vi "Request API.vi"(8 "error in (no error)":errorcluster, 10 "Promise":refnum<class "Promise.lvclass">, 11 "API Provider in":refnum<class "API Provider.lvclass">) -> (0 "error out":errorcluster, 3 "API Provider out":refnum<class "API Provider.lvclass">)   [LabVIEW 2020, in "Volatus.lvlib" / "API Provider.lvclass"]
uses:
  API Provider.lvclass
  lv-promises/Promises/Promise/Promise.lvclass
  ApiValue/ApiValue.lvclass
  C:/dev/lv20CE/relink/lv-promises/Promises/Value/Value.lvclass
  C:/dev/lv20CE/relink/lv-volatus/Volatus/ApiValue/ApiValue.lvclass
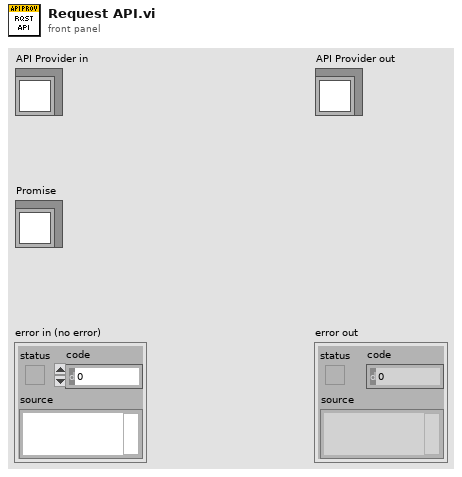
[diagram p1: front panel]
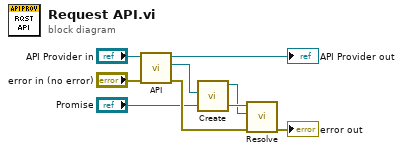
[diagram p0: block diagram]
diagram:
  n1 = call-dynamic "API.vi"("error in (no error)"="error in (no error)", "API Provider in"="API Provider in") -> ("error out"=w8:errorcluster, "API"=w3:refnum<class "API.lvclass">, "API Provider out"=→"API Provider out":refnum<class "API Provider.lvclass">)  [unwired: 7 in]
  n2 = call "Create.vi"("API"=w3) -> ("ApiValue out"=w2:refnum<class "ApiValue.lvclass">)  [unwired: 10 in]
  n3 = call "Resolve.vi"("error in (no error)"=w8, "Result"=w2, "Promise in"="Promise") -> ("error out"=→"error out":errorcluster)  [unwired: 7 in, 1 out]
